vi "MQTT_ConnAck_Read.vi"(8 "error in (no error)":errorcluster, 11 "connection ID":refnum<k5>) -> (0 "error out":errorcluster, 1 "QoS Level":T2, 2 "Connection Status":T1=enum."Connection refused: not authorized", 3 "connection ID out":refnum<k5>, 5 "MessageType":T3)   [LabVIEW 2025, in "DAQIO MQTT.lvlib"]
doc: "This VI processes the connection acknowledge message from the server.\n\n© 2015 - daq.io, LLC - Peter Adelhardt"
uses:
  DAQIO MQTT.lvlib
  Controls/MessageType.ctl
  Controls/QoS.ctl
  Controls/Connection_Return_Codes.ctl
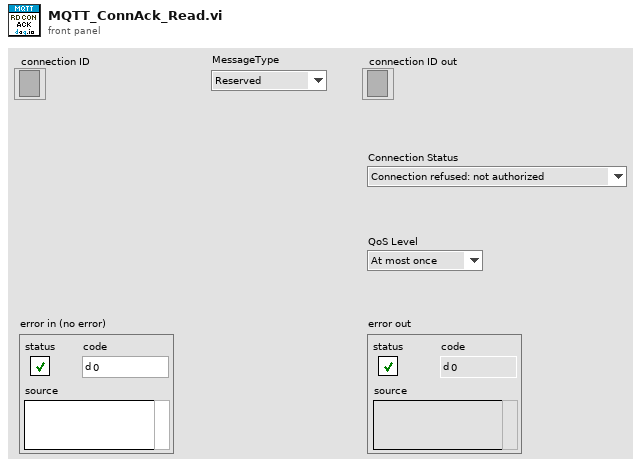
[diagram p1: front panel]
types:
  T1 = typedef "DAQIO MQTT.lvlib/Connection_Return_Codes.ctl" = enum16{"Connection accepted", "Connection refused: unacceptable protocol version", "Connection refused: identifier rejected", "Connection refused: Server unavailable", "Connection refused: bad user name or password", "Connection refused: not authorized"}
  T2 = typedef "DAQIO MQTT.lvlib/QoS.ctl" = enum8{"At most once", "At least once", "Exactly once", "Reserved"}
  T3 = typedef "DAQIO MQTT.lvlib/MessageType.ctl" = enum32{"Reserved", "CONNECT", "CONNACK", "PUBLISH", "PUBACK", "PUBREC", "PUBREL", "PUBCOMP", "SUBSCRIBE", "SUBACK", "UNSUBSCRIBE", "UNSUBACK", "PINGREQ", "PINGRESP", "DISCONNECT", "Reserved2"}
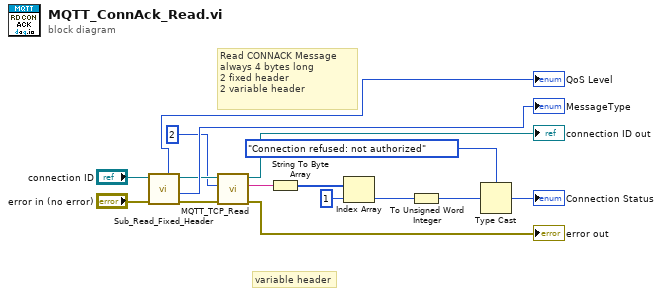
[diagram p0: block diagram]
diagram:
  # "variable header"
  # "Read CONNACK Message\nalways 4 bytes long\n2 fixed header\n2 variable header"
  n1 = call "Sub_Read_Fixed_Header.vi"("error in (no error)"="error in (no error)", "connection ID"="connection ID") -> ("error out"=w5:errorcluster, "MessageType"=→"MessageType":T3, "connection ID out"=w6:refnum<k5>, "QoS Level"=→"QoS Level":T2)  [unwired: 3 in, 3 out]
  n2 = call "MQTT_TCP_Read.vi"("error in (no error)"=w5, "bytes to read"=2, "connection ID"=w6) -> ("error out"=→"error out":errorcluster, "data out"=w3:string, "connection ID out"=→"connection ID out":refnum<k5>)  [unwired: 6 in]
  n3 = String To Byte Array(string=w3) -> (unsigned byte array=w2:u8[])
  n4 = Index Array(array=w2, index=1) -> (element=w9:u8)
  n5 = To Unsigned Word Integer(number=w9) -> (unsigned 16bit integer=w1:u16)
  n6 = Type Cast(type=Connection_Return_Codes."Connection refused: not authorized" ("Conn Return Code"), x=w1) -> (*(type *) &x=→"Connection Status":T1)
